vi "SerialCycle.vi"   [LabVIEW 2019]
uses:
  02 Mode/SerialMode/SerialClass.lvclass
types:
  T1 = typedef "串口枚举.ctl" = enum16{"ini", "增", "删", "查", "改"}
  T2 = typedef "SerialData.ctl" = cluster{"VISA串口名称":refnum<visa-resource-name>, "波特率":u32, "停止位":u16, "流控制":u16, "数据位":u16, "奇偶校验":enum16{"None", "Odd", "Even", "Mark", "Space"}, "超时":u32, "启用终止符？":bool, "终止符":u8}
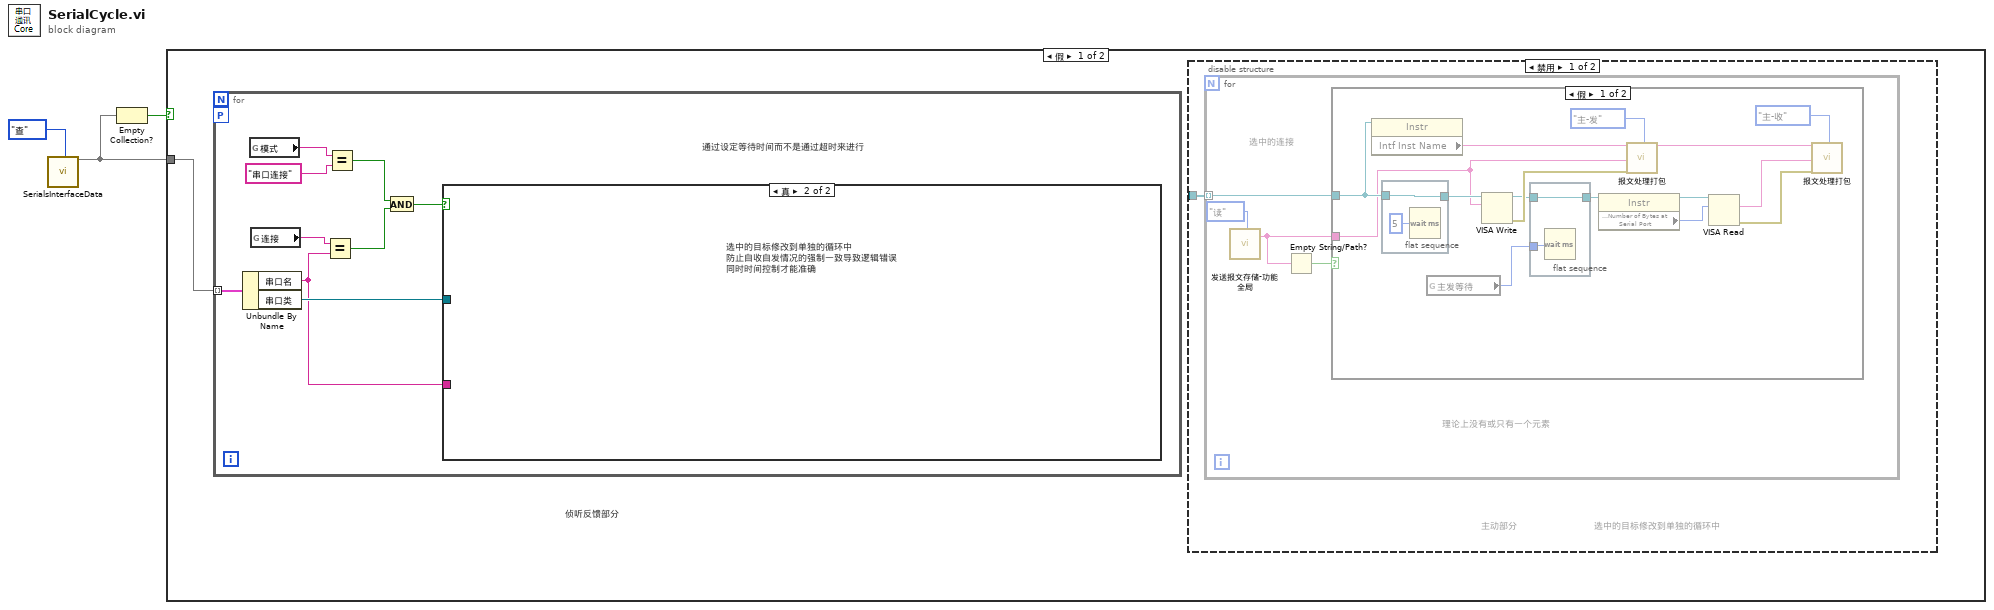
[diagram p0: block diagram]
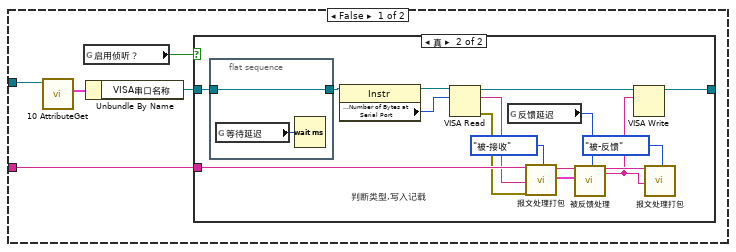
[diagram p4: hidden frame]
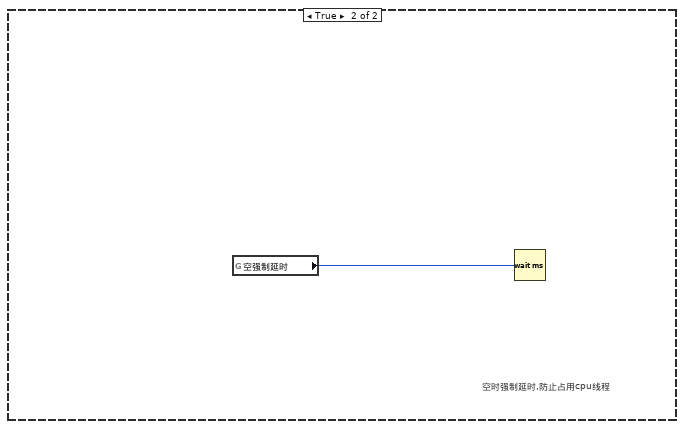
[diagram p6: hidden frame]
diagram:
  n1 = call "SerialsInterfaceData.vi"("串口枚举"=串口枚举."查") -> ("串口表"=w2:map{string, refnum<class "SerialClass.lvclass">})  [unwired: 17 in, 1 out]
  n2 = Empty Collection?(1:w2) -> (0:w3:bool)
  n3 = case shown="假" w3 {
    tunnel: w2 -> [w4 _]
    frame False {
      # "侦听反馈部分"
      n4 = for {
        tunnel: w4 -> [w37] mode=indexing
        workers-P: _ -> [_]
        # "通过设定等待时间而不是通过超时来进行"
        n5 = Unbundle By Name(w37) -> ("串口名"=w30:string, "串口类"=w36:refnum<class "SerialClass.lvclass">)
        n6 = global read "全局-配置识别.vi" "模式"() -> (w35:string)
        n7 = global read "全局-配置识别.vi" "连接"() -> (w33:string)
        n8 = Equal?(x=w33, y=w30) -> (x = y?=w31:bool)
        n9 = Equal?(x=w35, y="串口连接") -> (x = y?=w32:bool)
        n10 = And(x=w32, y=w31) -> (x .and. y?=w29:bool)
        n11 = case shown="真" w29 {
          tunnel: w36 -> [w42 _]
          tunnel: w30 -> [w39 _]
          frame False {
            n12 = call-dynamic "10 AttributeGet.vi"("SerialClass 输入"=w42) -> ("串口配置"=w41:T2)  [unwired: 7 in, 3 out]
            n13 = global read "全局-被反馈配置.vi" "启用侦听？"() -> (w38:bool)
            n14 = Unbundle By Name(w41) -> ("VISA串口名称"=w40:refnum<visa-resource-name>)
            n15 = case shown="真" w38 {
              tunnel: w40 -> [w43 w44]
              tunnel: w39 -> [_ w57]
              tunnel: [w43 w52] -> _
              frame False {
              }
              frame True {
                # "判断类型,写入记载"
                n16 = flat-sequence {
                  tunnel: [w61] -> w45
                  tunnel: w44 -> [w61]
                  frame #0 {
                    n17 = global read "全局-配置识别.vi" "等待延迟"() -> (w60:u32)
                    n18 = Wait (ms)(milliseconds to wait=w60) -> ()  [unwired: 1 out]
                  }
                }
                n19 = property class="Instr"(reference=w45) -> (reference out=w59:refnum<visa-resource-name>, "Serial Settings:Number of Bytes at Serial Port"=w58:u32)  [unwired: 1 in, 1 out]
                n20 = VISA Read(VISA resource name=w59, byte count=w58) -> (VISA resource name out=w54:refnum<visa-resource-name>, read buffer=w56:string, error out=w53:errorcluster)  [unwired: 1 in, 1 out]
                n21 = global read "全局-配置识别.vi" "反馈延迟"() -> (w46:u32)
                n22 = call "报文处理打包.vi"("识别名称"=w57, "报文"=w56, "Error In"=w53, "类型"=enum16{"被-接收", "被-反馈", "主-发", "主-收"}."被-接收") -> ("识别名称输出"=w51:string, "被收校验信息"=w50:cluster{"可用？":bool, "功能码":u8, "无crc报文":u8[]})  [unwired: 14 in]
                n23 = call "被反馈处理.vi"("识别名称"=w51, "校验信息"=w50, "等待时间（毫秒）"=w46) -> ("识别名称输出"=w49:string, "反馈"=w48:string)  [unwired: 15 in]
                n24 = VISA Write(VISA resource name=w54, write buffer=w48) -> (VISA resource name out=w52:refnum<visa-resource-name>)  [unwired: 1 in, 2 out]
                n25 = call "报文处理打包.vi"("识别名称"=w49, "报文"=w48, "类型"=enum16{"被-接收", "被-反馈", "主-发", "主-收"}."被-反馈") -> ()  [unwired: 15 in, 2 out]
              }
            }
          }
          frame True {
            # "选中的目标修改到单独的循环中\n防止自收自发情况的强制一致导致逻辑错误\n同时时间控制才能准确"
          }
        }
      }
      n26 = disable-structure shown="禁用" {
        disable-tunnel: _ -> [w5 _]
        frame Disabled {
          # "选中的目标修改到单独的循环中"
          # "主动部分"
          n27 = for {
            tunnel: w5 -> [w9] mode=indexing
            # "选中的连接"
            # "理论上没有或只有一个元素"
            n28 = call "发送报文存储-功能全局.vi"("枚举"=enum16{"ini", "读", "写"}."读") -> ("报文输出"=w6:string)  [unwired: 18 in]
            n29 = Empty String/Path?(string/path=w6) -> (empty?=w7:bool)
            n30 = case shown="假" w7 {
              tunnel: w9 -> [w21 _]
              tunnel: w6 -> [w15 _]
              frame False {
                n31 = property class="Instr"(reference=w21) -> ("Intf Inst Name"=w17:string)  [unwired: 1 in, 2 out]
                n32 = flat-sequence {
                  tunnel: [w27] -> w24
                  tunnel: w21 -> [w27]
                  frame #0 {
                    n33 = Wait (ms)(milliseconds to wait=u32 5 ("等待时间（毫秒）")) -> ()  [unwired: 1 out]
                  }
                }
                n34 = global read "全局-配置识别.vi" "主发等待"() -> (w10:u32)
                n35 = VISA Write(VISA resource name=w24, write buffer=w15) -> (VISA resource name out=w12:refnum<visa-resource-name>, error out=w13:errorcluster)  [unwired: 1 in, 1 out]
                n36 = flat-sequence {
                  tunnel: w12 -> [w26]
                  tunnel: [w26] -> w11
                  tunnel: w10 -> [w25]
                  frame #0 {
                    n37 = Wait (ms)(milliseconds to wait=w25) -> ()  [unwired: 1 out]
                  }
                }
                n38 = property class="Instr"(reference=w11) -> (reference out=w22:refnum<visa-resource-name>, "Serial Settings:Number of Bytes at Serial Port"=w23:u32)  [unwired: 1 in, 1 out]
                n39 = call "报文处理打包.vi"("识别名称"=w17, "报文"=w15, "Error In"=w13, "类型"=enum16{"被-接收", "被-反馈", "主-发", "主-收"}."主-发") -> ("识别名称输出"=w16:string)  [unwired: 14 in, 1 out]
                n40 = VISA Read(VISA resource name=w22, byte count=w23) -> (read buffer=w18:string, error out=w14:errorcluster)  [unwired: 1 in, 2 out]
                n41 = call "报文处理打包.vi"("识别名称"=w16, "报文"=w18, "Error In"=w14, "类型"=enum16{"被-接收", "被-反馈", "主-发", "主-收"}."主-收") -> ()  [unwired: 14 in, 2 out]
              }
              frame True {
              }
            }
          }
        }
        frame Enabled {
        }
      }
    }
    frame True {
      # "空时强制延时,防止占用cpu线程"
      n42 = global read "全局-配置识别.vi" "空强制延时"() -> (w62:u32)
      n43 = Wait (ms)(milliseconds to wait=w62) -> ()  [unwired: 1 out]
    }
  }
